vi "High_Voltage_Power_Supply_Control.vi"() -> ()   [LabVIEW 2017]
uses:
  High_Voltage_Power_Supply_Control_States.ctl
panel:
  out "CH1 AND CH2 \n  CURRENTS":T1(graph)
  in  "File Path (.csv)":path
  out "CH1 AND CH2 \n   VOLTAGES":T2(graph)
  in  "STOP (T = stop)":bool
  in  "COM Port In":refnum<visa-resource-name>
  in  "Measuring speed (s)":dbl=1.0 caption="Time Target (s)" min=0.0
  out "Emergency Stop (T = active)":bool
  out "Connection (T = active)":bool
  in  "Control Mode (T = CV, F = CC)":bool=TRUE
  out "CH2 CURRENT OUT (mA)":dbl format="%.2f"
  out "CH2 VOLTAGE OUT (V)":i32
  out "CH1 CURRENT OUT (mA)":dbl format="%.2f"
  out "CH1 VOLTAGE OUT (V)":i32
  in  "CH2 CURRENT SET (0...5 mA)":dbl=5.0 min=0.0 max=5.0 step=0.1 format="%_4f"
  in  "CH1 CURRENT SET (0...5 mA)":dbl=5.0 min=0.0 max=5.0 step=0.1 format="%_4f"
  in  "CH2 VOLTAGE SET (0...+2000 V)":i16 min=0 max=2000 step=100
  in  "CH1 VOLTAGE SET (-2000...0 V)":i16 min=-2000 max=0 step=100
  in  "CH2 ON/OFF (T = ON)":bool
  in  "CH1 ON/OFF (T = ON)":bool
  # "High Voltage Power Supply"
  # "CH1: -2000...0 V"
  # "CH2: 0...+2000 V"
  # "Save voltages and currents in CSV file"
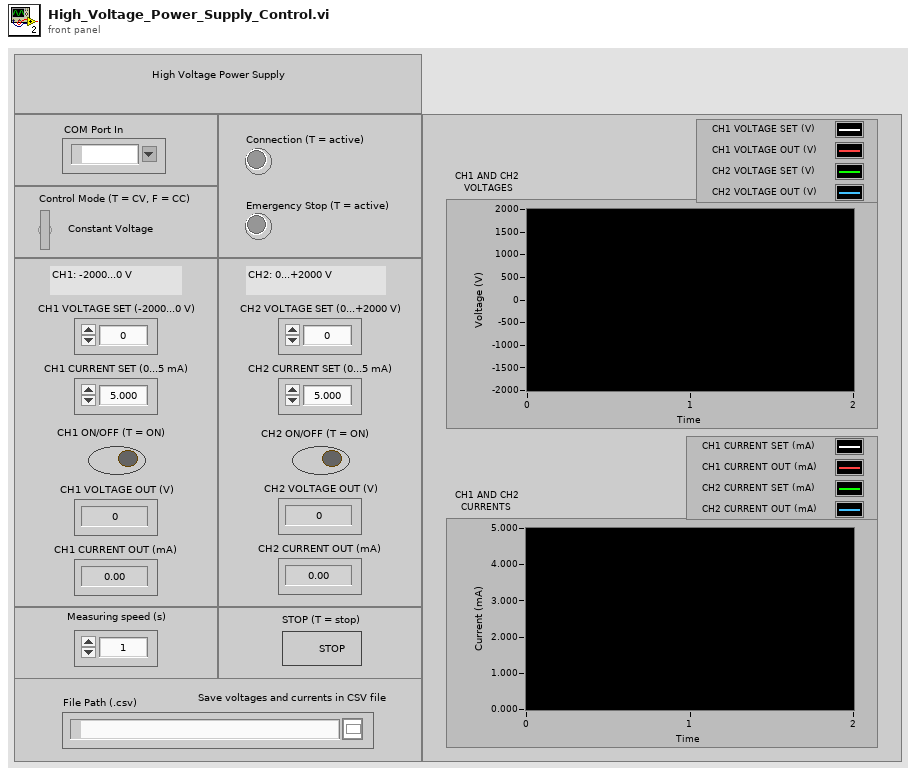
[diagram p1: front panel]
types:
  T1 = cluster{"Value":dbl, "Value":dbl, "Value":dbl, "Value":dbl}
  T2 = cluster{"Value":i16, "Value":i32, "Value":i16, "Value":i32}
  T3 = typedef "High_Voltage_Power_Supply_Control_States.ctl" = enum16{"CONTROL", "STOP", "INITIALISATION"}
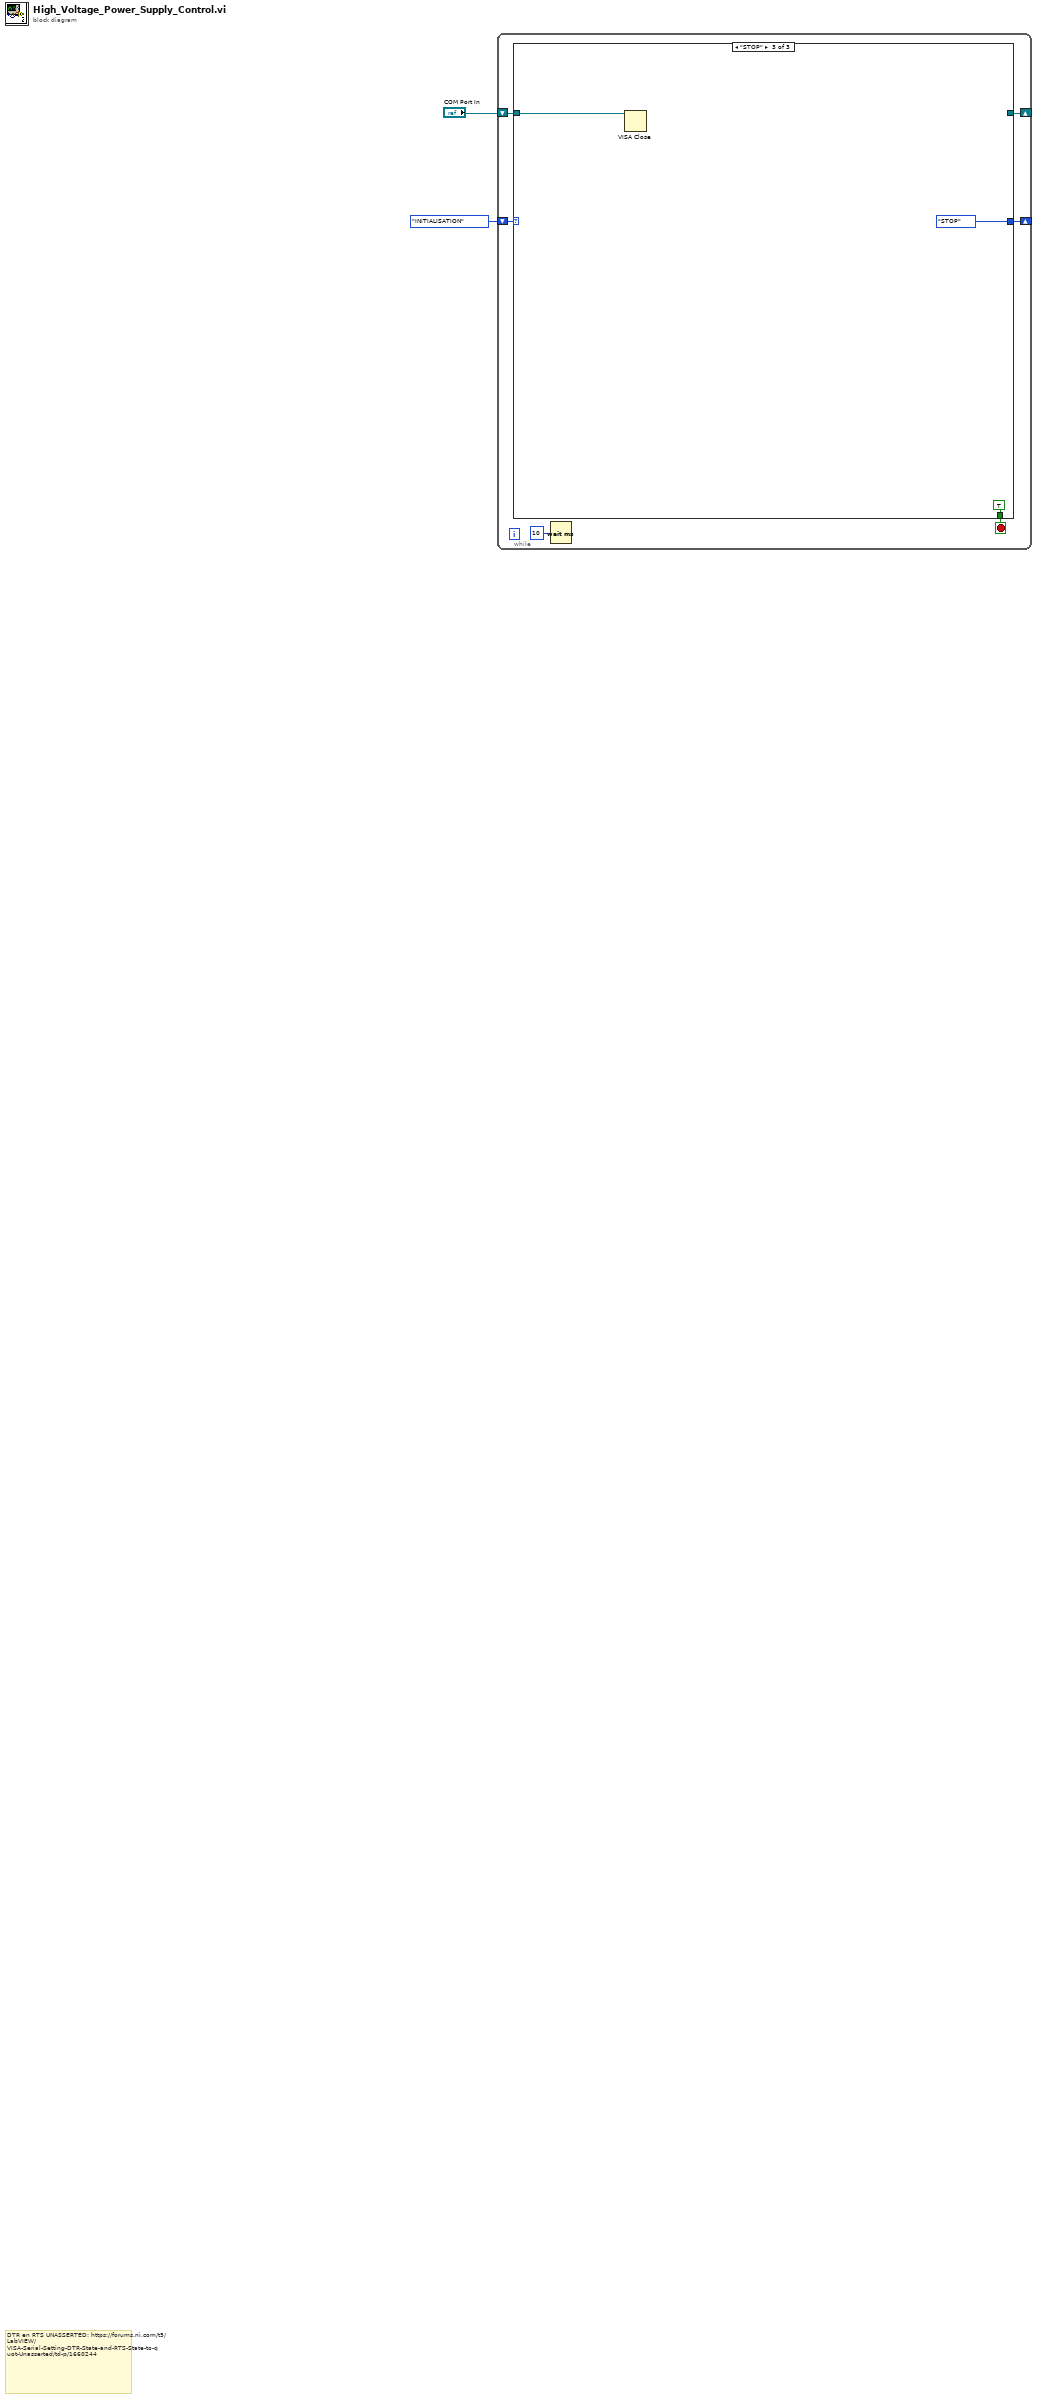
[diagram p0: block diagram]
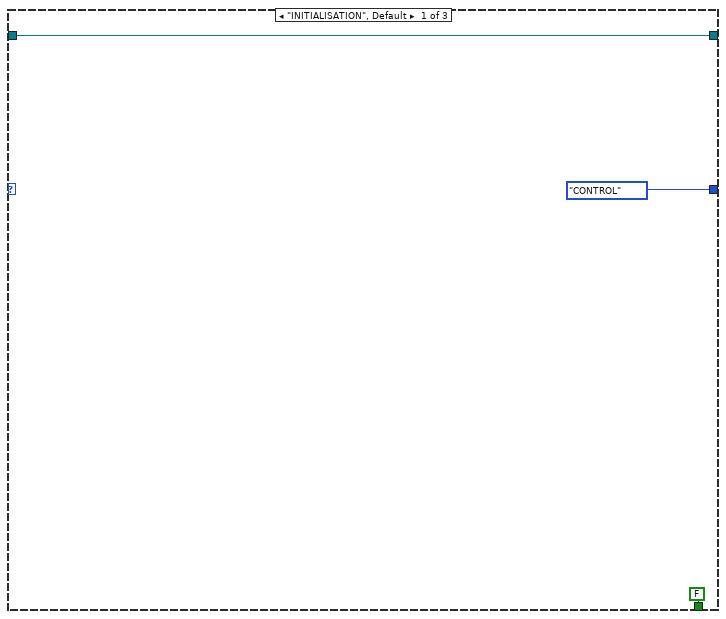
[diagram p2: hidden frame]
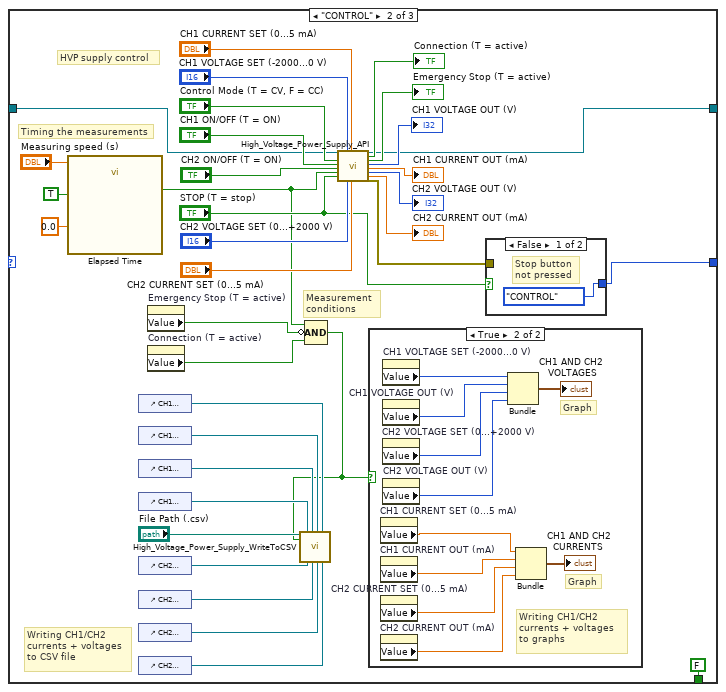
[diagram p3: hidden frame]
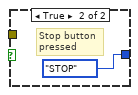
[diagram p5: hidden frame]
diagram:
  # "DTR en RTS UNASSERTED: https://forums.ni.com/t5/LabVIEW/VISA-Serial-Setting-DTR-State-and-RTS-State-to-quot-Unasserted/td-p/1660244"
  n1 = while {
    shift-right: [w6] -> _
    shift-left: High_Voltage_Power_Supply_Control_States."INITIALISATION" -> [w7]
    shift-right: [w4] -> _
    shift-left: "COM Port In" -> [w3]
    stop <- w5 stop-if-true
    n2 = case shown="\"STOP\"" w7 {
      tunnel: w3 -> [w9 w15 w61]
      tunnel: [High_Voltage_Power_Supply_Control_States."CONTROL" w45 High_Voltage_Power_Supply_Control_States."STOP"] -> w6
      tunnel: [FALSE FALSE TRUE] -> w5
      tunnel: [w9 w17 _] -> w4
      frame "INITIALISATION", Default {
      }
      frame "CONTROL" {
        # "Measurement \nconditions"
        # "Writing CH1/CH2 currents + voltages to CSV file"
        # "Timing the measurements"
        # "HVP supply control"
        n3 = call "Elapsed Time"("Time Target (s)"="Measuring speed (s)", "Auto Reset"=TRUE, "Set Start Time (s)"=0.0) -> ("Time has Elapsed"=w13:bool)  [unwired: 9 in, 7 out]
        n4 = control-ref of="CH1 CURRENT OUT (mA)"() -> (w23:refnum<vi>)
        n5 = control-ref of="CH1 VOLTAGE OUT (V)"() -> (w24:refnum<vi>)
        n6 = control-ref of="CH1 CURRENT SET (0...5 mA)"() -> (w25:refnum<vi>)
        n7 = control-ref of="CH1 VOLTAGE SET (-2000...0 V)"() -> (w26:refnum<vi>)
        n8 = control-ref of="CH2 VOLTAGE SET (0...+2000 V)"() -> (w22:refnum<vi>)
        n9 = control-ref of="CH2 CURRENT SET (0...5 mA)"() -> (w21:refnum<vi>)
        n10 = control-ref of="CH2 VOLTAGE OUT (V)"() -> (w20:refnum<vi>)
        n11 = control-ref of="CH2 CURRENT OUT (mA)"() -> (w19:refnum<vi>)
        n12 = property on="Emergency Stop (T = active)" class="Bool (strict)"() -> ("Value"=w12:bool)  [unwired: 2 in, 2 out]
        n13 = property on="Connection (T = active)" class="Bool (strict)"() -> ("Value"=w14:bool)  [unwired: 2 in, 2 out]
        n14 = Compound Arithmetic op=AND(w13, invert w12, w14) -> (w16:bool)
        n15 = call "High_Voltage_Power_Supply_WriteToCSV.vi"("File Path (.csv)"="File Path (.csv)", "WriteToCSV (T = write)"=w16, "CH1 VOLTAGE SET (V)"=w26, "CH2 VOLTAGE SET (V)"=w22, "CH1 CURRENT SET (mA)"=w25, "CH2 CURRENT SET (mA)"=w21, "CH1 VOLTAGE OUT (V)"=w24, "CH2 VOLTAGE OUT (V)"=w20, "CH1 CURRENT OUT (mA)"=w23, "CH2 CURRENT OUT (mA)"=w19) -> ()  [unwired: 9 in, 1 out]
        n16 = call "High_Voltage_Power_Supply_API.vi"("COM Port In"=w15, "Control Mode (T = CV, F = CC)"="Control Mode (T = CV, F = CC)", "CH1 ON/OFF (T = ON)"="CH1 ON/OFF (T = ON)", "CH2 ON/OFF (T = ON)"="CH2 ON/OFF (T = ON)", "MEASURE (T = measure)"=w13, "STOP (T = stop)"="STOP (T = stop)", "CH1 VOLTAGE SET (-2000...0 V)"="CH1 VOLTAGE SET (-2000...0 V)", "CH2 VOLTAGE SET (0...+2000 V)"="CH2 VOLTAGE SET (0...+2000 V)", "CH1 CURRENT SET (0...5 mA)"="CH1 CURRENT SET (0...5 mA)", "CH2 CURRENT SET (0...5 mA)"="CH2 CURRENT SET (0...5 mA)") -> ("COM Port Out"=w17:refnum<visa-resource-name>, "Connection (T = active)"=→"Connection (T = active)":bool, "Emergency Stop (T = active)"=→"Emergency Stop (T = active)":bool, "CH1 VOLTAGE OUT (V)"=→"CH1 VOLTAGE OUT (V)":i32, "CH1 CURRENT OUT (mA)"=→"CH1 CURRENT OUT (mA)":dbl, "CH2 VOLTAGE OUT (V)"=→"CH2 VOLTAGE OUT (V)":i32, "CH2 CURRENT OUT (mA)"=→"CH2 CURRENT OUT (mA)":dbl, "error out"=w46:errorcluster)  [unwired: 10 in]
        n17 = case shown="True" w16 {
          frame False {
            # "No measurements are written to charts"
          }
          frame True {
            # "Graph"
            # "Graph"
            # "Writing CH1/CH2 currents + voltages to graphs"
            n18 = property on="CH1 CURRENT SET (0...5 mA)" class="DigNum (strict)"() -> ("Value"=w51:dbl)  [unwired: 2 in, 2 out]
            n19 = property on="CH1 CURRENT OUT (mA)" class="DigNum (strict)"() -> ("Value"=w50:dbl)  [unwired: 2 in, 2 out]
            n20 = property on="CH2 CURRENT SET (0...5 mA)" class="DigNum (strict)"() -> ("Value"=w49:dbl)  [unwired: 2 in, 2 out]
            n21 = property on="CH2 CURRENT OUT (mA)" class="DigNum (strict)"() -> ("Value"=w48:dbl)  [unwired: 2 in, 2 out]
            n22 = property on="CH1 VOLTAGE SET (-2000...0 V)" class="DigNum (strict)"() -> ("Value"=w55:i16)  [unwired: 2 in, 2 out]
            n23 = property on="CH1 VOLTAGE OUT (V)" class="DigNum (strict)"() -> ("Value"=w56:i32)  [unwired: 2 in, 2 out]
            n24 = property on="CH2 VOLTAGE SET (0...+2000 V)" class="DigNum (strict)"() -> ("Value"=w53:i16)  [unwired: 2 in, 2 out]
            n25 = property on="CH2 VOLTAGE OUT (V)" class="DigNum (strict)"() -> ("Value"=w52:i32)  [unwired: 2 in, 2 out]
            n26 = Bundle("Value"=w55, "Value"=w56, "Value"=w53, "Value"=w52) -> (→"CH1 AND CH2 \n   VOLTAGES":T2)  [unwired: 1 in]
            n27 = Bundle("Value"=w51, "Value"=w50, "Value"=w49, "Value"=w48) -> (→"CH1 AND CH2 \n  CURRENTS":T1)  [unwired: 1 in]
          }
        }
        n28 = case shown="False" "STOP (T = stop)" {
          tunnel: w46 -> [_ _]
          tunnel: [High_Voltage_Power_Supply_Control_States."CONTROL" High_Voltage_Power_Supply_Control_States."STOP"] -> w45
          frame False {
            # "Stop button\nnot pressed"
          }
          frame True {
            # "Stop button\npressed"
          }
        }
      }
      frame "STOP" {
        n29 = VISA Close(VISA resource name=w61) -> ()  [unwired: 1 in, 1 out]
      }
    }
    n30 = Wait (ms)(milliseconds to wait=u32 10) -> ()  [unwired: 1 out]
  }
